vi "GlobalDriveJoysticks.vi"() -> ()   [LabVIEW 2020]
panel:
  in  "Middle Button":bool
  in  "Z":dbl
  in  "Y":dbl
  in  "X":dbl
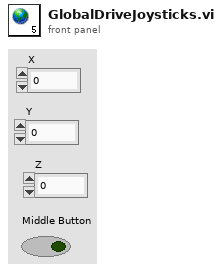
[diagram p1: front panel]
diagram:
